vi "coords_degree_to_dec.vi"(1 "Seconds":string, 2 "Minutes":string, 3 "Degrees":string) -> (0 "Decimal":dbl)   [LabVIEW 2015]
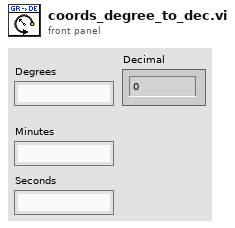
[diagram p1: front panel]
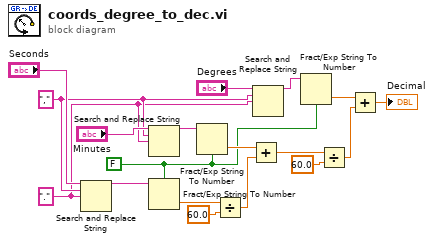
[diagram p0: block diagram]
diagram:
  w1 = "." ("replace string (\"\")")
  w2 = "," ("search string")
  w9 = FALSE ("use system decimal point (T)")
  n1 = Search and Replace String(input string="Seconds", search string=w2, replace string=w1) -> (result string=w7:string)  [unwired: 5 in, 3 out]
  n2 = Search and Replace String(input string="Minutes", search string=w2, replace string=w1) -> (result string=w5:string)  [unwired: 5 in, 3 out]
  n3 = Fract/Exp String To Number(use system decimal point (T)=w9, string=w7) -> (number=w12:dbl)  [unwired: 2 in, 1 out]
  n4 = Fract/Exp String To Number(use system decimal point (T)=w9, string=w5) -> (number=w11:dbl)  [unwired: 2 in, 1 out]
  n5 = Divide(x=w12, y=60.0) -> (x/y=w15:dbl)
  n6 = Add(x=w11, y=w15) -> (x+y=w16:dbl)
  n7 = Search and Replace String(input string="Degrees", search string=w2, replace string=w1) -> (result string=w3:string)  [unwired: 5 in, 3 out]
  n8 = Fract/Exp String To Number(use system decimal point (T)=w9, string=w3) -> (number=w10:dbl)  [unwired: 2 in, 1 out]
  n9 = Divide(x=w16, y=60.0) -> (x/y=w14:dbl)
  n10 = Add(x=w10, y=w14) -> (x+y=→"Decimal":dbl)
